vi "Strip Path__ogtk.vi"   [LabVIEW 2020]
doc: "Functions identically to LabVIEW \"Strip Path\" function, but is polymorphic to also allow the path input to be an array. If an array is used, the outputs become arrays."
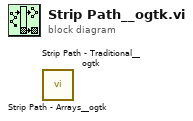
[diagram p0: block diagram]
diagram:
  n1 = call <userlib>:"Strip Path - Arrays__ogtk.vi"() -> ()  [unwired: 1 in, 2 out]
  n2 = call <userlib>:"Strip Path - Traditional__ogtk.vi"() -> ()  [unwired: 1 in, 2 out]
